vi "select region to get floor piece.vi"(11 "type":enum16{"Z", "I", "O", "S", "L", "J", "T", "N"}(ring)) -> ()   [LabVIEW 2018]
uses:
  vision/vision info 2.vi
panel:
  out "needed":bool
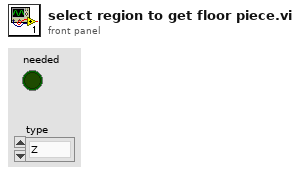
[diagram p1: front panel]
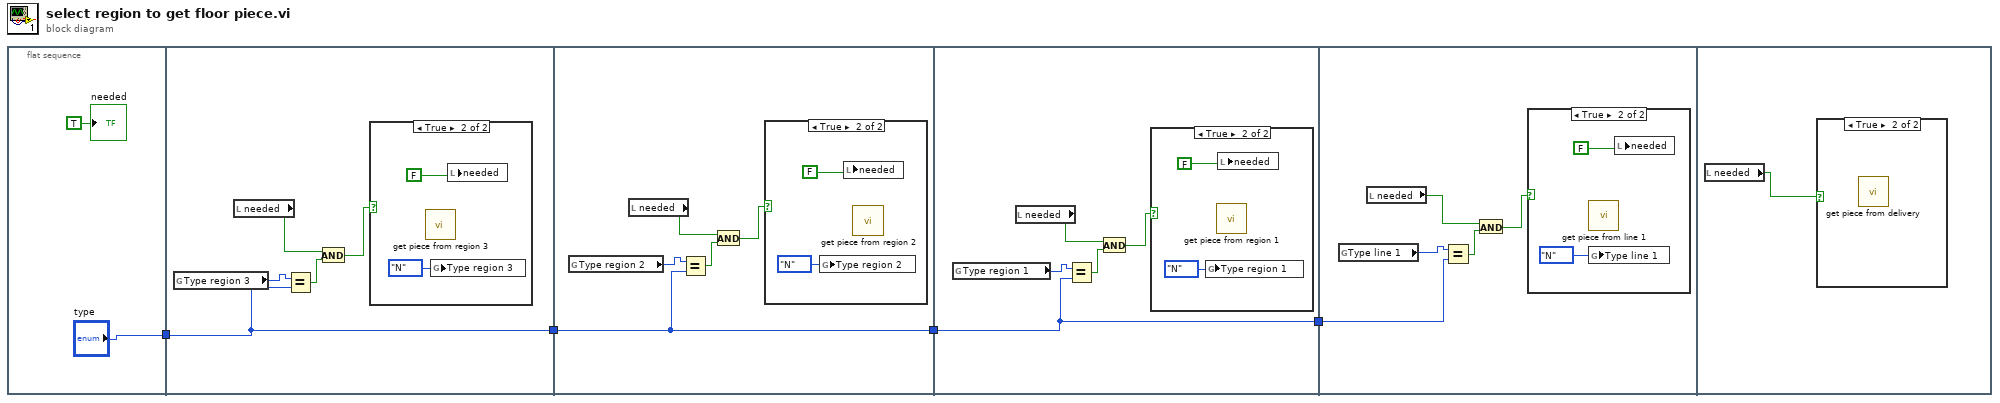
[diagram p0: block diagram]
diagram:
  n1 = flat-sequence {
    tunnel: ["type"] -> w4
    tunnel: w4 -> [w7]
    tunnel: [w7] -> w3
    tunnel: w3 -> [w14]
    tunnel: [w14] -> w2
    tunnel: w2 -> [w21]
    tunnel: [w21] -> w1
    tunnel: w1 -> [w28]
    frame #0 {
      "needed" <- TRUE ("taken")
    }
    frame #1 {
      n2 = global read "vision info 2.vi" "Type region 3"() -> (w11:enum16{"Z", "I", "O", "S", "L", "J", "T", "N"})
      n3 = local read "needed"() -> (w9:bool)
      n4 = Equal?(x=w11, y=w7) -> (x = y?=w10:bool)
      n5 = And(x=w9, y=w10) -> (x .and. y?=w8:bool)
      n6 = case shown="True" w8 {
        frame False {
        }
        frame True {
          n7 = call "get piece from region 3.vi"() -> ()  [unwired: 12 in]
          n8 = global write "vision info 2.vi" "Type region 3"(enum16{"Z", "I", "O", "S", "L", "J", "T", "N"}."N" ("Type region 3")) -> ()
          n9 = local write "needed"(FALSE ("taken")) -> ()
        }
      }
    }
    frame #2 {
      n10 = global read "vision info 2.vi" "Type region 2"() -> (w18:enum16{"Z", "I", "O", "S", "L", "J", "T", "N"})
      n11 = local read "needed"() -> (w16:bool)
      n12 = Equal?(x=w18, y=w14) -> (x = y?=w17:bool)
      n13 = And(x=w16, y=w17) -> (x .and. y?=w15:bool)
      n14 = case shown="True" w15 {
        frame False {
        }
        frame True {
          n15 = global write "vision info 2.vi" "Type region 2"(enum16{"Z", "I", "O", "S", "L", "J", "T", "N"}."N" ("Type region 3")) -> ()
          n16 = local write "needed"(FALSE ("taken")) -> ()
          n17 = call "get piece from region 2.vi"() -> ()  [unwired: 12 in]
        }
      }
    }
    frame #3 {
      n18 = global read "vision info 2.vi" "Type region 1"() -> (w25:enum16{"Z", "I", "O", "S", "L", "J", "T", "N"})
      n19 = local read "needed"() -> (w23:bool)
      n20 = Equal?(x=w25, y=w21) -> (x = y?=w24:bool)
      n21 = And(x=w23, y=w24) -> (x .and. y?=w22:bool)
      n22 = case shown="True" w22 {
        frame False {
        }
        frame True {
          n23 = global write "vision info 2.vi" "Type region 1"(enum16{"Z", "I", "O", "S", "L", "J", "T", "N"}."N" ("Type region 3")) -> ()
          n24 = call "get piece from region 1.vi"() -> ()  [unwired: 12 in]
          n25 = local write "needed"(FALSE ("taken")) -> ()
        }
      }
    }
    frame #4 {
      n26 = global read "vision info 2.vi" "Type line 1"() -> (w32:enum16{"Z", "I", "O", "S", "L", "J", "T", "N"})
      n27 = local read "needed"() -> (w30:bool)
      n28 = Equal?(x=w32, y=w28) -> (x = y?=w31:bool)
      n29 = And(x=w30, y=w31) -> (x .and. y?=w29:bool)
      n30 = case shown="True" w29 {
        frame False {
        }
        frame True {
          n31 = call "get piece from line 1.vi"() -> ()  [unwired: 12 in]
          n32 = global write "vision info 2.vi" "Type line 1"(enum16{"Z", "I", "O", "S", "L", "J", "T", "N"}."N" ("Type region 3")) -> ()
          n33 = local write "needed"(FALSE ("taken")) -> ()
        }
      }
    }
    frame #5 {
      n34 = local read "needed"() -> (w35:bool)
      n35 = case shown="True" w35 {
        frame False {
        }
        frame True {
          n36 = call "get piece from delivery.vi"() -> ()  [unwired: 12 in]
        }
      }
    }
  }
